vi "Remove Default connection.vi"(0 "vi reference":refnum<vi>, 11 "error in (no error)":errorcluster) -> (4 "vi reference out":refnum<vi>, 15 "error out":errorcluster)   [LabVIEW 2021, in "Migrator.lvlib"]
uses:
  Migrator.lvlib
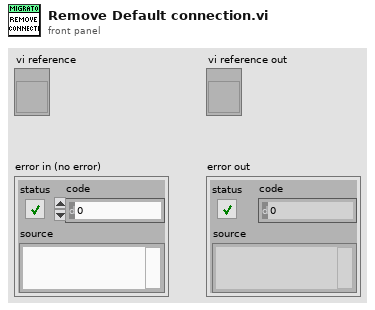
[diagram p1: front panel]
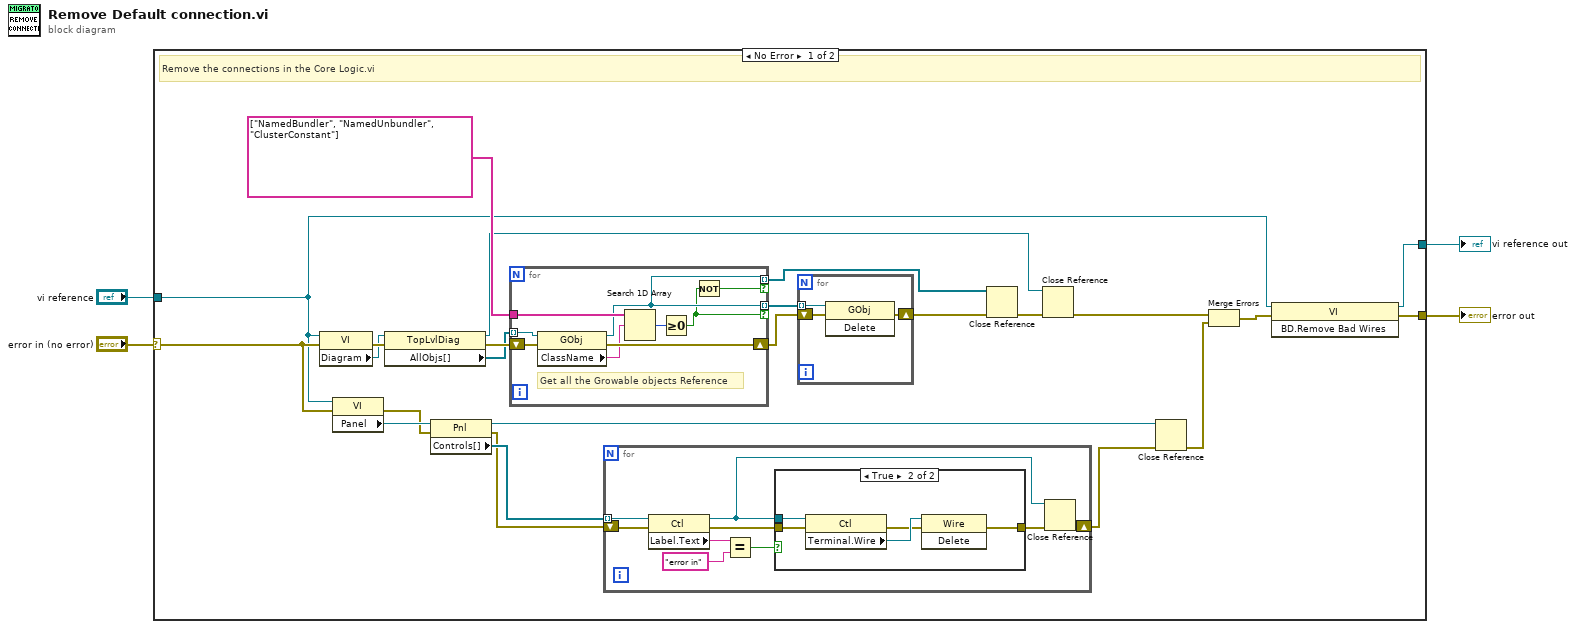
[diagram p0: block diagram]
diagram:
  n1 = case shown="No Error" "error in (no error)" {
    selector: "error in (no error)" -> [w10 w57]
    tunnel: [w7 w57] -> w4
    tunnel: "vi reference" -> [w8 w56]
    tunnel: [w6 w56] -> w1
    frame No Error {
      # "Remove the connections in the Core Logic.vi"
      n2 = property class="VI"(reference=w8, error in=w10) -> (error out=w27:errorcluster, "Diagram"=w19:refnum<vi>)  [unwired: 1 out]
      n3 = property class="VI"(reference=w8, error in=w10) -> (error out=w16:errorcluster, "Panel"=w18:refnum<vi>)  [unwired: 1 out]
      n4 = property class="TopLvlDiag"(reference=w19, error in=w27) -> (reference out=w9:refnum<vi>, error out=w24:errorcluster, "AllObjs[]"=w20:refnum<vi>[])
      n5 = property class="Pnl"(reference=w18, error in=w16) -> (reference out=w14:refnum<vi>, error out=w15:errorcluster, "Controls[]"=w17:refnum<vi>[])
      n6 = for {
        tunnel: w20 -> [w51] mode=indexing
        tunnel: string[] ["NamedBundler", "NamedUnbundler", "ClusterConstant"] -> [w54]
        tunnel: [w49] -> w25 mode=indexing if=w48
        tunnel: [w49] -> w5 mode=indexing if=w47
        shift-right: [w52] -> w23
        shift-left: w24 -> [w53]
        # "Get all the Growable objects Reference"
        n7 = property class="GObj"(reference=w51, error in=w53) -> (reference out=w49:refnum<vi>, error out=w52:errorcluster, "ClassName"=w50:string)
        n8 = Search 1D Array(1D array=w54, element=w50) -> (index of element=w55:i32)  [unwired: 1 in]
        n9 = Greater Or Equal To 0?(x=w55) -> (x >= 0?=w48:bool)
        n10 = Not(x=w48) -> (.not. x?=w47:bool)
      }
      n11 = for {
        tunnel: w17 -> [w37] mode=indexing
        shift-right: [w29] -> w13
        shift-left: w15 -> [w33]
        n12 = property class="Ctl"(reference=w37, error in=w33) -> (reference out=w31:refnum<vi>, error out=w32:errorcluster, "Label.Text"=w36:string)
        n13 = Equal?(x=w36, y="error in") -> (x = y?=w34:bool)
        n14 = case shown="True" w34 {
          tunnel: w31 -> [_ w43]
          tunnel: w32 -> [w38 w40]
          tunnel: [w38 w39] -> w30
          frame False {
          }
          frame True {
            n15 = property class="Ctl"(reference=w43, error in=w40) -> (error out=w41:errorcluster, "Terminal.Wire"=w42:refnum<vi>)  [unwired: 1 out]
            n16 = invoke class="Wire" method="Delete"(reference=w42, error in=w41) -> (error out=w39:errorcluster)  [unwired: 1 in, 2 out]
          }
        }
        n17 = Close Reference(reference=w31, error in (no error)=w30) -> (error out=w29:errorcluster)
      }
      n18 = for {
        tunnel: w25 -> [w46] mode=indexing
        shift-right: [w44] -> w22
        shift-left: w23 -> [w45]
        n19 = invoke class="GObj" method="Delete"(reference=w46, error in=w45) -> (error out=w44:errorcluster)  [unwired: 1 in, 2 out]
      }
      n20 = Close Reference(reference=w5, error in (no error)=w22) -> (error out=w26:errorcluster)
      n21 = Close Reference(reference=w9, error in (no error)=w26) -> (error out=w21:errorcluster)
      n22 = Close Reference(reference=w14, error in (no error)=w13) -> (error out=w11:errorcluster)
      n23 = Merge Errors(w21, w11) -> (w12:errorcluster)
      n24 = invoke class="VI" method="BD.Remove Bad Wires"(reference=w8, error in=w12) -> (reference out=w6:refnum<vi>, error out=w7:errorcluster)  [unwired: 1 in, 1 out]
    }
    frame Error {
    }
  }
  "error out" <- w4
  "vi reference out" <- w1
